vi "QuerrySQL.vi"(8 "error in (no error)":errorcluster, 10 "Jsonconfig":string, 11 "String":string) -> (0 "error out":errorcluster, 3 "Array":string[][](array[string]))   [LabVIEW 2015]
uses:
  Libraries/lv_mysql_connector_v1_lv8/typedefs/mysql_authentication.ctl
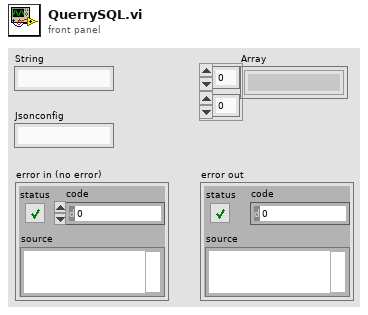
[diagram p1: front panel]
types:
  T1 = typedef "mysql_authentication.ctl" = cluster{"User":string, "Password":string, "Database":string}
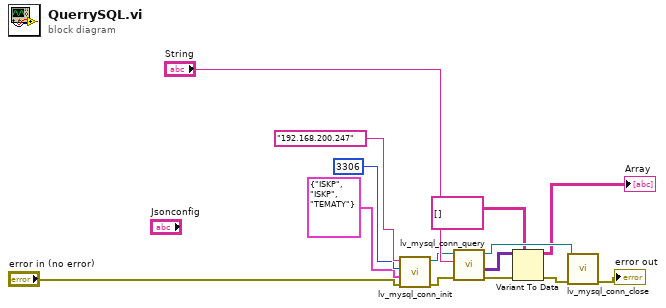
[diagram p0: block diagram]
diagram:
  n1 = call "lv_mysql_conn_init.vi"("error in (no error)"="error in (no error)", "Authentication"=T1 {"User"="ISKP", "Password"="ISKP", "Database"="TEMATY"}, "Port"=u16 3306, "IP Address"="192.168.200.247") -> ("error out"=w14:errorcluster, "connection ID out"=w12:refnum<k5>)  [unwired: 6 in]
  n2 = call "lv_mysql_conn_query.vi"("error in (no error)"=w14, "Query"="String", "connection ID"=w12) -> ("error out"=w3:errorcluster, "Return Data"=w7:variant[][], "connection ID out"=w6:refnum<k5>)  [unwired: 5 in, 1 out]
  n3 = Variant To Data(error in=w3, type=string[][] [], Variant=w7) -> (data=→"Array":string[][], error out=w4:errorcluster)
  n4 = call "lv_mysql_conn_close.vi"("error in (no error)"=w4, "connection ID"=w6) -> ("error out"=→"error out":errorcluster)  [unwired: 9 in]
